vi "Receiver_2.vi"() -> ()   [LabVIEW 2013]
uses:
  <vilib>/imath/engines/lvmath/Plug In/_Char/NIMS_CH_character datatype.ctl
  <vilib>/imath/engines/lvmath2/RunTimeEngine/ErrorHandling/NIMS_Finalize Error.vi
  <vilib>/imath/engines/lvmath2/RunTimeEngine/Managers/WorkSpace/UID Generator.vi
  <vilib>/imath/engines/lvmath2/RunTimeEngine/Managers/SymbolTable/Clear UID.vi
  <vilib>/imath/engines/lvmath2/RunTimeEngine/NodeEndStatement/NIMS_NodeEndStatement_Output.vi
  <instcachedir>/0/NIMS_NodeEndStatement_Output_53EC0D466D134D7ABD903AC30B43404B.lvgen/NIMS_NodeEndStatement_Output_53EC0D466D134D7ABD903AC30B43404B_000.vi
  <instcachedir>/0/NIMS_NodeEndStatement_Output_53EC0D466D134D7ABD903AC30B43404B.lvgen/NIMS_NodeEndStatement_Output_53EC0D466D134D7ABD903AC30B43404B_011.vi
  <vilib>/imath/engines/lvmath2/RunTimeEngine/BuiltInFunctions/close/NIMS_close(Enums).vi
  <vilib>/imath/engines/lvmath2/RunTimeEngine/BuiltInFunctions/numelements/NIMS_numelements.vi
  <instcachedir>/0/NIMS_numelements_A776DA77F73142F68C2F209B523114C5.lvgen/NIMS_numelements_A776DA77F73142F68C2F209B523114C5_001.vi
  LabVIEW Data/MathScriptVIs/MCStatic_31879994332_4a1719067c7d5a83f01437ef7afed563.vi
  <instcachedir>/0/MCStatic_31879994332_4a1719067c7d5a83f01437ef7afed563_B552334F5E31422DA0051DD0B7CE2B4C.lvgen/MCStatic_31879994332_4a1719067c7d5a83f01437ef7afed563_B552334F5E31422DA0051DD0B7CE2B4C_000.vi
  <vilib>/imath/engines/lvmath2/RunTimeEngine/BuiltInFunctions/figure/NIMS_figure(I32).vi
  <vilib>/imathl/engines/lvmath/Functions/Error Handling/Create Error.vi
  <vilib>/imath/engines/lvmath/Plug In/_Char/NIMS_CH_Character RV to String.vi
  <vilib>/imath/engines/lvmath2/RunTimeEngine/BuiltInFunctions/plot/NIMS_plot(G, Str).vi
  <instcachedir>/0/NIMS_plot(G, Str)_30D49D8623E0484DBD39D394DDFCBE95.lvgen/NIMS_plot(G, Str)_30D49D8623E0484DBD39D394DDFCBE95_005.vi
  <vilib>/imath/engines/lvmath2/RunTimeEngine/BuiltInFunctions/title/NIMS_title.vi
  LabVIEW Data/MathScriptVIs/MCStatic_31879994332_366ffe5655d941eb3ff0cfc563e39803.vi
  <instcachedir>/0/MCStatic_31879994332_366ffe5655d941eb3ff0cfc563e39803_D7DA22716DE04C8BBFF6AC70E7C1861D.lvgen/MCStatic_31879994332_366ffe5655d941eb3ff0cfc563e39803_D7DA22716DE04C8BBFF6AC70E7C1861D_000.vi
  <instcachedir>/0/NIMS_numelements_A776DA77F73142F68C2F209B523114C5.lvgen/NIMS_numelements_A776DA77F73142F68C2F209B523114C5_003.vi
  <vilib>/imath/engines/lvmath/Plug In/_Char/NIMS_CH_Character 1D to U8 1D.vi
  <vilib>/imath/engines/lvmath2/RunTimeEngine/BuiltInFunctions/plot/NIMS_plot(G, Arb).vi
  <instcachedir>/0/NIMS_plot(G, Arb)_C3943409FB664E118D06A85D9C4CA97C.lvgen/NIMS_plot(G, Arb)_C3943409FB664E118D06A85D9C4CA97C_000.vi
  <vilib>/imath/engines/lvmath2/RunTimeEngine/BuiltInFunctions/hold/NIMS_hold(Enums).vi
  <vilib>/imath/engines/lvmath2/RunTimeEngine/BuiltInFunctions/imag/NIMS_imag(Complex).vi
  <instcachedir>/0/NIMS_imag(Complex)_3180D40D00C843A49C2B33397F857BF3.lvgen/NIMS_imag(Complex)_3180D40D00C843A49C2B33397F857BF3_002.vi
  LabVIEW Data/MathScriptVIs/MCStatic_31879994332_6309011b735c7d3bdc345e9dbe068425.vi
  <instcachedir>/0/MCStatic_31879994332_6309011b735c7d3bdc345e9dbe068425_079E241E9A4346CA9D2DFB9112E326FB.lvgen/MCStatic_31879994332_6309011b735c7d3bdc345e9dbe068425_079E241E9A4346CA9D2DFB9112E326FB_000.vi
  LabVIEW Data/MathScriptVIs/MCStatic_31879994332_e0c6d33342fcfeb52dca76011519375f.vi
  <instcachedir>/0/MCStatic_31879994332_e0c6d33342fcfeb52dca76011519375f_339AF80C0AAC43069D5B64E593FFC926.lvgen/MCStatic_31879994332_e0c6d33342fcfeb52dca76011519375f_339AF80C0AAC43069D5B64E593FFC926_000.vi
  <vilib>/imath/engines/lvmath2/RunTimeEngine/IndexRead/NIMS V(R2).vi
  <instcachedir>/0/NIMS V(R2)_C76619605A0E4E9F8B2FA9389712AC47.lvgen/NIMS V(R2)_C76619605A0E4E9F8B2FA9389712AC47_000.vi
  <vilib>/imath/engines/lvmath2/RunTimeEngine/ArithmeticOperatorToken/NIMS_ArithmeticOperator_plus.vi
  <instcachedir>/0/NIMS_ArithmeticOperator_plus_8A46DAFC24D445C9B2C97B626139369E.lvgen/NIMS_ArithmeticOperator_plus_8A46DAFC24D445C9B2C97B626139369E_005.vi
  <instcachedir>/0/NIMS_plot(G, Str)_30D49D8623E0484DBD39D394DDFCBE95.lvgen/NIMS_plot(G, Str)_30D49D8623E0484DBD39D394DDFCBE95_001.vi
  <vilib>/imath/engines/lvmath2/RunTimeEngine/ErrorHandling/NIMS_Create Error From Enums.vi
  <vilib>/imath/engines/lvmath2/RunTimeEngine/BuiltInFunctions/grid/NIMS_grid(Enums).vi
  <vilib>/imath/engines/lvmath2/RunTimeEngine/VariableToken/NIMS_VariableToken_CondDefined.vi
  <instcachedir>/0/NIMS_VariableToken_CondDefined_9DC5CEC47F8146B087FA2781C705B229.lvgen/NIMS_VariableToken_CondDefined_9DC5CEC47F8146B087FA2781C705B229_003.vi
  <vilib>/imath/engines/lvmath/Functions/Error Handling/MergeErrorsWrapper.vi
  <instcachedir>/0/NIMS_NodeEndStatement_Output_53EC0D466D134D7ABD903AC30B43404B.lvgen/NIMS_NodeEndStatement_Output_53EC0D466D134D7ABD903AC30B43404B_001.vi
  <vilib>/imath/engines/lvmath2/RunTimeEngine/RunTimeType/NIMS_RunTimeType_From StrictType (excl LVString).vi
  <instcachedir>/0/NIMS_RunTimeType_From StrictType (excl LVString)_4DEE718D6EB74582AA20236969C084FC.lvgen/NIMS_RunTimeType_From StrictType (excl LVString)_4DEE718D6EB74582AA20236969C084FC_000.vi
  <vilib>/imath/engines/lvmath2/RunTimeEngine/LocalVariableDefStatement/MC_LocalVariableDefStatement_Display.vi
  <vilib>/imath/engines/lvmath2/RunTimeEngine/BuiltInFunctions/linramp/NIMS_linramp.vi
  <vilib>/imath/engines/lvmath2/RunTimeEngine/BuiltInFunctions/abs/NIMS_abs(signed).vi
  <instcachedir>/0/NIMS_abs(signed)_C4FCB8E6058B49B797C7C8D53CA5F6EC.lvgen/NIMS_abs(signed)_C4FCB8E6058B49B797C7C8D53CA5F6EC_006.vi
  <vilib>/imath/engines/lvmath2/RunTimeEngine/BuiltInFunctions/max/1 input/NIMS_max(RV).vi
  <instcachedir>/0/NIMS_max(RV)_237633DB1D604D5BA7001287DF3C7957.lvgen/NIMS_max(RV)_237633DB1D604D5BA7001287DF3C7957_000.vi
  <vilib>/imath/engines/lvmath2/RunTimeEngine/BuiltInFunctions/zeros/NIMS_V=zeros(I32,I32).vi
  <vilib>/imath/engines/lvmath2/RunTimeEngine/RangeToken/NIMS_Range_R2 - Integer.vi
  <instcachedir>/0/NIMS_Range_R2 - Integer_C51C130E5EA5464EA148B28CDAB9615A.lvgen/NIMS_Range_R2 - Integer_C51C130E5EA5464EA148B28CDAB9615A_000.vi
  <vilib>/imath/engines/lvmath2/RunTimeEngine/CommandStatement/MC_CommandStatement_break.vi
  <vilib>/imath/engines/lvmath2/RunTimeEngine/IndexRead/NIMS V(S).vi
  <instcachedir>/0/NIMS V(S)_0488751826AF41519A22953C041130DC.lvgen/NIMS V(S)_0488751826AF41519A22953C041130DC_005.vi
  <instcachedir>/0/NIMS_abs(signed)_C4FCB8E6058B49B797C7C8D53CA5F6EC.lvgen/NIMS_abs(signed)_C4FCB8E6058B49B797C7C8D53CA5F6EC_002.vi
  LabVIEW Data/MathScriptVIs/MCStatic_31879994332_56053b3087a32285ab019b20dd55a053.vi
  <instcachedir>/0/MCStatic_31879994332_56053b3087a32285ab019b20dd55a053_ABD68300304F468FBDE6379C6945ADEA.lvgen/MCStatic_31879994332_56053b3087a32285ab019b20dd55a053_ABD68300304F468FBDE6379C6945ADEA_000.vi
  <vilib>/imath/engines/lvmath2/RunTimeEngine/IndexReplace/NIMS V(S)=S.vi
  <instcachedir>/0/NIMS V(S)=S_66A18068148B4981A312229A93EA5C06.lvgen/NIMS V(S)=S_66A18068148B4981A312229A93EA5C06_001.vi
  LabVIEW Data/MathScriptVIs/MCStatic_31879994332_59775c3ea1da542a74dd2e471b583196.vi
  <instcachedir>/0/MCStatic_31879994332_59775c3ea1da542a74dd2e471b583196_003FAE1D6247465EB97E783626A83D88.lvgen/MCStatic_31879994332_59775c3ea1da542a74dd2e471b583196_003FAE1D6247465EB97E783626A83D88_001.vi
  <instcachedir>/0/NIMS V(S)=S_66A18068148B4981A312229A93EA5C06.lvgen/NIMS V(S)=S_66A18068148B4981A312229A93EA5C06_000.vi
  <instcachedir>/0/NIMS V(R2)_C76619605A0E4E9F8B2FA9389712AC47.lvgen/NIMS V(R2)_C76619605A0E4E9F8B2FA9389712AC47_001.vi
  <instcachedir>/0/NIMS V(S)_0488751826AF41519A22953C041130DC.lvgen/NIMS V(S)_0488751826AF41519A22953C041130DC_000.vi
  <instcachedir>/0/NIMS_plot(G, Str)_30D49D8623E0484DBD39D394DDFCBE95.lvgen/NIMS_plot(G, Str)_30D49D8623E0484DBD39D394DDFCBE95_000.vi
  MATLAB_func/TX_RRC_filtering.m
  MATLAB_func/rtrcpulse.m
  MATLAB_func/b2_16qam.m
  MATLAB_func/RX_RRC_filtering.m
  MATLAB_func/gardner_symbol_recovery.m
  MATLAB_func/frequency_synchronisation_sample.m
  MATLAB_func/phase_synchronisation_sample.m
  <vilib>/imath/engines/lvmath2/RunTimeEngine/Managers/SymbolTable/NIMS_WorkSpace.lvlib
  <vilib>/Analysis/NI_AALBase.lvlib
panel:
  in  "Numeric":dbl
  out "L":i32
  out "Symbols 4":cdb[](graph)
  out "wave array":cdb[](array[numeric])
  out "Symbols 3":cdb[](graph)
  out "Waveform Chart":dbl[](graph)
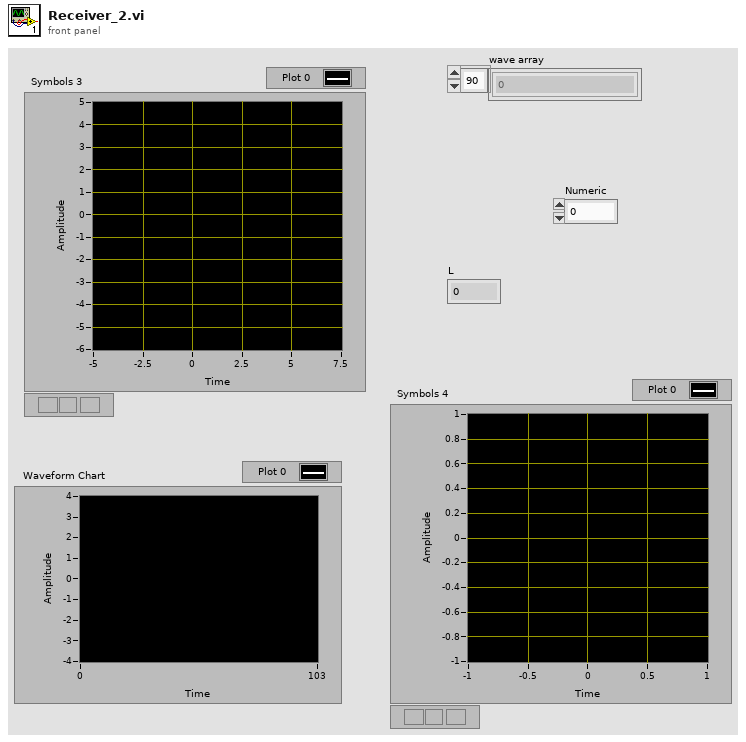
[diagram p1: front panel]
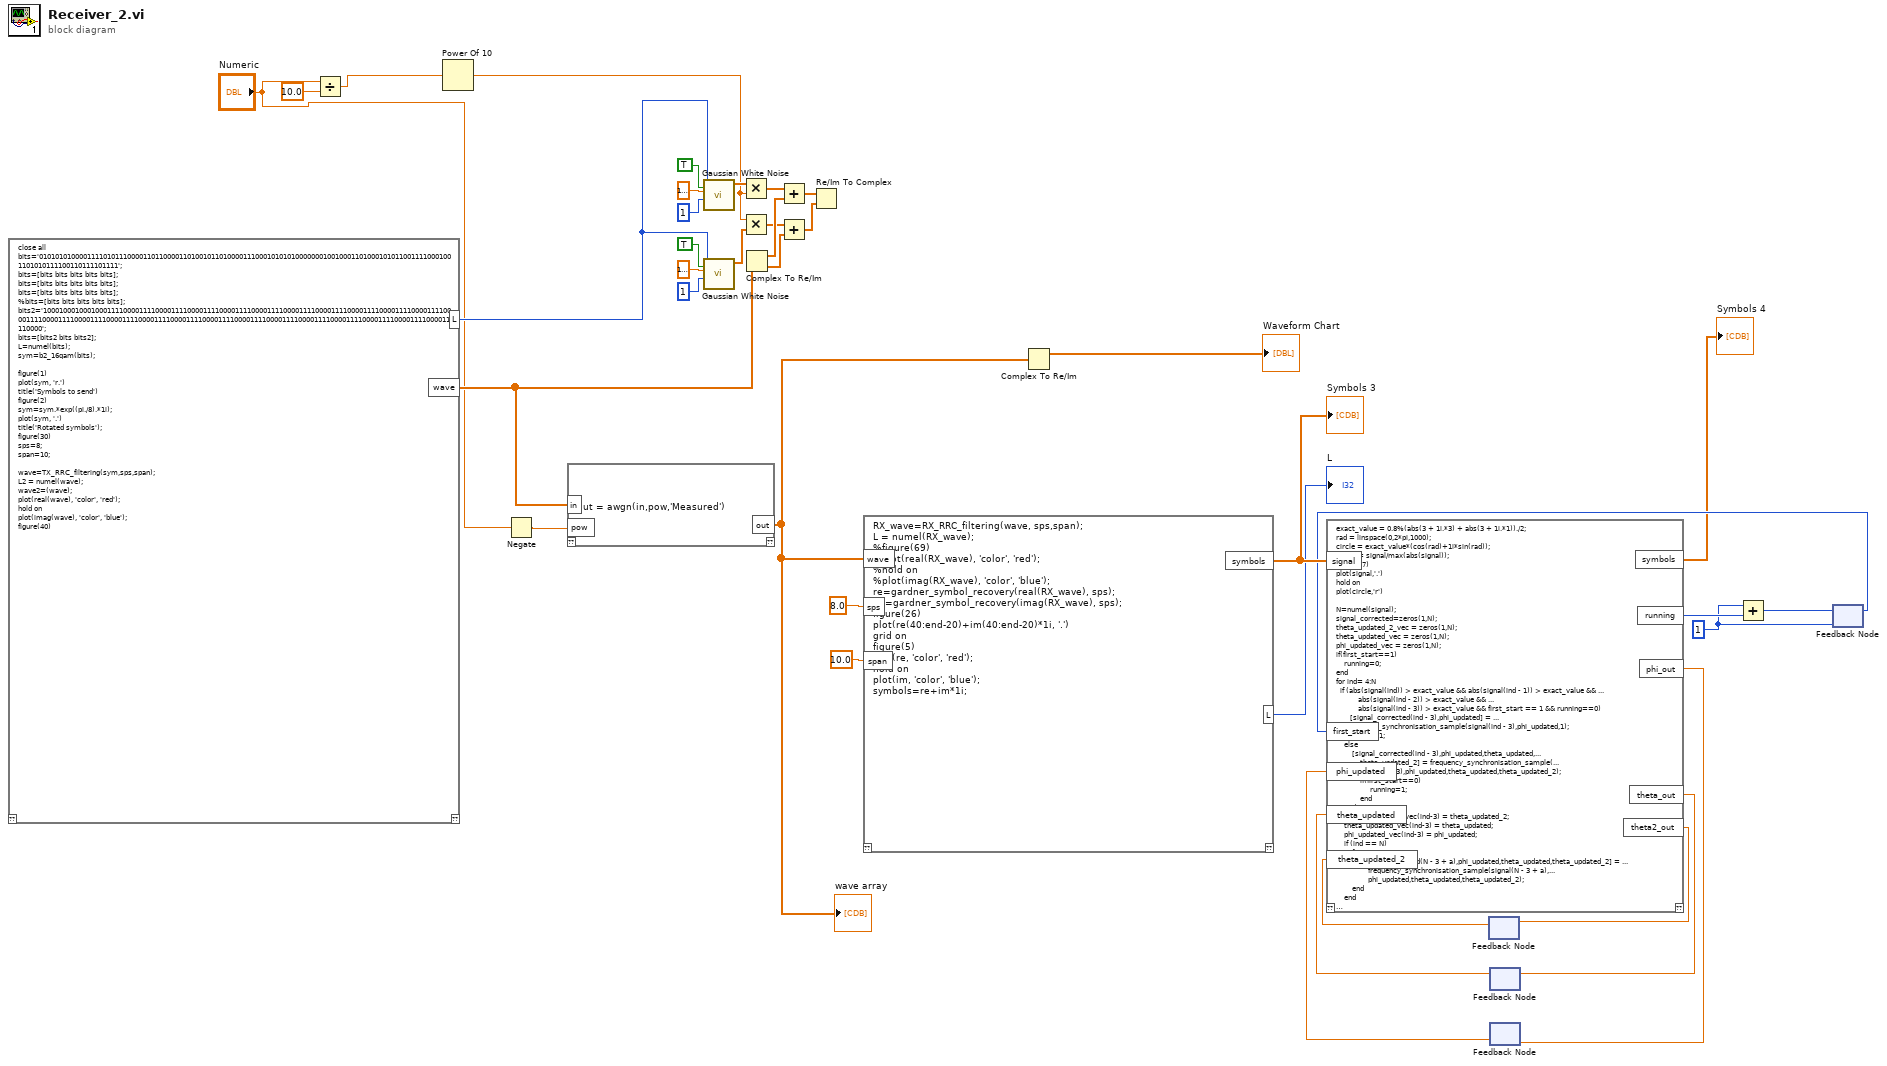
[diagram p0: block diagram]
diagram:
  w26 = 1 ("x")
  n1 = mathscript code="close all\nbits='01010101000011110101110000110110000110100101101000011100010101010000000100100011010001010110011110001001101010111100110111101111';\nbits=[bits bits bits bits bits];\nbits=[bits bits bits bits bits];\nbits=[bits bits bits bits bits];\n%bits=[bits bits bits bits bits];\nbits2='100010001000100011110000111100001111000011110000111100001111000011110000111100001111000011110000111100001111000011110000111100001111000011110000111100001111000011110000111100001111000011110000111100001111000011110000';\nbits=[bits2 bits bits2];\nL=numel(bits);\nsym=b2_16qam(bits);\n\nfigure(1)\nplot(sym, 'r.')\ntitle('Symbols to send')\nfigure(2)\nsym=sym.*exp((pi./8).*1i);\nplot(sym, '.')\ntitle('Rotated symbols');\nfigure(30)\nsps=8;\nspan=10;\n\nwave=TX_RRC_filtering(sym,sps,span);\nL2 = numel(wave);\nwave2=(wave);\nplot(real(wave), 'color', 'red');\nhold on\nplot(imag(wave), 'color', 'blue');\nfigure(40)"() -> ("L"=w16:i32, "wave"=w5:cdb[])  [unwired: 1 in, 1 out]
  n2 = Divide(x="Numeric", y=10.0) -> (x/y=w3:dbl)
  n3 = Power Of 10(x=w3) -> (10^x=w7:dbl)
  n4 = Negate(x="Numeric") -> (-x=w1:dbl)
  n5 = script code="out = awgn(in,pow,'Measured')"("in"=w5, "pow"=w1) -> ("out"=w4:cdb[])  [unwired: 1 in, 1 out]
  "wave array" <- w4
  n6 = call <vilib>:"Gaussian White Noise.vi"("initialize?"=TRUE, "seed"=1, "standard deviation"=1.0000000000000002, "samples"=w16) -> ("Gaussian noise pattern"=w11:dbl[])  [unwired: 6 in, 1 out]
  n7 = call <vilib>:"Gaussian White Noise.vi"("initialize?"=TRUE, "seed"=1, "standard deviation"=1.0000000000000002, "samples"=w16) -> ("Gaussian noise pattern"=w8:dbl[])  [unwired: 6 in, 1 out]
  n8 = Multiply(x=w11, y=w7) -> (x*y=w10:dbl[])
  n9 = Multiply(x=w7, y=w8) -> (x*y=w9:dbl[])
  n10 = Complex To Re/Im(x + iy=w5) -> (x=w12:dbl[], y=w15:dbl[])
  n11 = Add(x=w10, y=w12) -> (x+y=w13:dbl[])
  n12 = Add(x=w9, y=w15) -> (x+y=w14:dbl[])
  n13 = Re/Im To Complex(1:w14, 2:w13) -> ()  [unwired: 1 out]
  n14 = mathscript code="RX_wave=RX_RRC_filtering(wave, sps,span);\nL = numel(RX_wave);\n%figure(69)\n%plot(real(RX_wave), 'color', 'red');\n%hold on\n%plot(imag(RX_wave), 'color', 'blue');\nre=gardner_symbol_recovery(real(RX_wave), sps);\nim=gardner_symbol_recovery(imag(RX_wave), sps);\nfigure(26)\nplot(re(40:end-20)+im(40:end-20)*1i, '.')\ngrid on\nfigure(5)\nplot(re, 'color', 'red');\nhold on\nplot(im, 'color', 'blue');\nsymbols=re+im*1i;"("wave"=w4, "sps"=8.0, "span"=10.0) -> ("symbols"=w35:cdb[], "L"=→"L":i32)  [unwired: 1 in, 1 out]
  "Symbols 3" <- w35
  n15 = Complex To Re/Im(x + iy=w4) -> (x=→"Waveform Chart":dbl[])  [unwired: 1 out]
  n16 = feedback #1() -> (w31:dbl)  [unwired: 1 in]
  n17 = feedback #2() -> (w33:dbl)  [unwired: 1 in]
  n18 = feedback #3() -> (w29:dbl)  [unwired: 1 in]
  n19 = feedback #4(w26) -> (w25:i32)
  n20 = mathscript code="exact_value = 0.8%(abs(3 + 1i.*3) + abs(3 + 1i.*1))./2;\nrad = linspace(0,2*pi,1000);\ncircle = exact_value*(cos(rad)+1i*sin(rad));\nsignal = signal/max(abs(signal));\nfigure(17)\nplot(signal,'.')\nhold on\nplot(circle,'r')\n\nN=numel(signal);\nsignal_corrected=zeros(1,N);\ntheta_updated_2_vec = zeros(1,N);\ntheta_updated_vec = zeros(1,N);\nphi_updated_vec = zeros(1,N);\nif(first_start==1)\n    running=0;\nend\nfor ind= 4:N\n  if (abs(signal(ind)) > exact_value && abs(signal(ind - 1)) > exact_value && ...\n           abs(signal(ind - 2)) > exact_value && ...\n           abs(signal(ind - 3)) > exact_value && first_start == 1 && running==0)\n       [signal_corrected(ind - 3),phi_updated] = ...\n           phase_synchronisation_sample(signal(ind - 3),phi_updated,1);\n      running=1;\n    else\n        [signal_corrected(ind - 3),phi_updated,theta_updated,...\n            theta_updated_2] = frequency_synchronisation_sample(...\n            signal(ind-3),phi_updated,theta_updated,theta_updated_2);\n            if(first_start==0)\n                 running=1;\n            end\n    end\n    theta_updated_2_vec(ind-3) = theta_updated_2;\n    theta_updated_vec(ind-3) = theta_updated;\n    phi_updated_vec(ind-3) = phi_updated;\n    if (ind == N)\n        for a = 1:3\n            [signal_corrected(N - 3 + a),phi_updated,theta_updated,theta_updated_2] = ...\n                frequency_synchronisation_sample(signal(N - 3 + a),...\n                phi_updated,theta_updated,theta_updated_2);\n        end\n    end\n\nend\nfigure(28)\nplot(signal_corrected(1:end),'.')\nsymbols=signal_corrected;\nphi_out=phi_updated_vec(N-4);\ntheta_out=theta_updated_vec(N-5);\ntheta2_out=theta_updated_2_vec(N-4);\nfigure(8888)\nplot(theta_updated_2_vec)\ntitle('Accumulated frequency phase correction');\nfigure(479)\nplot(phi_updated_vec)\ntitle('Phase offset per symbol');\nhold off\nfigure(1337)\nplot(symbols(1000:end-20),'.')"("first_start"=w25, "signal"=w35, "phi_updated"=w29, "theta_updated"=w33, "theta_updated_2"=w31) -> ("symbols"=→"Symbols 4":cdb[], "running"=w28:i32, "phi_out"=w30:dbl, "theta2_out"=w32:dbl, "theta_out"=w34:dbl)  [unwired: 1 in, 1 out]
  n21 = feedback-in #1(w32) -> ()
  n22 = feedback-in #2(w34) -> ()
  n23 = feedback-in #3(w30) -> ()
  n24 = Add(x=w26, y=w28) -> (x+y=w27:i32)
  n25 = feedback-in #4(w27) -> ()
